vi "sync_issues.vi"(10 "CLZ Issues":string[][](array[string]), 11 "CV Issues":string[][](array[string])) -> (3 "Array":T1[](array[typedef]))   [LabVIEW 2024, in "CLZ_to_ComicVine.lvlib"]
uses:
  CLZ_to_ComicVine.lvlib
  typedefs/issue_match--cluster.ctl
  typedefs/clz_matching_issue--cluster.ctl
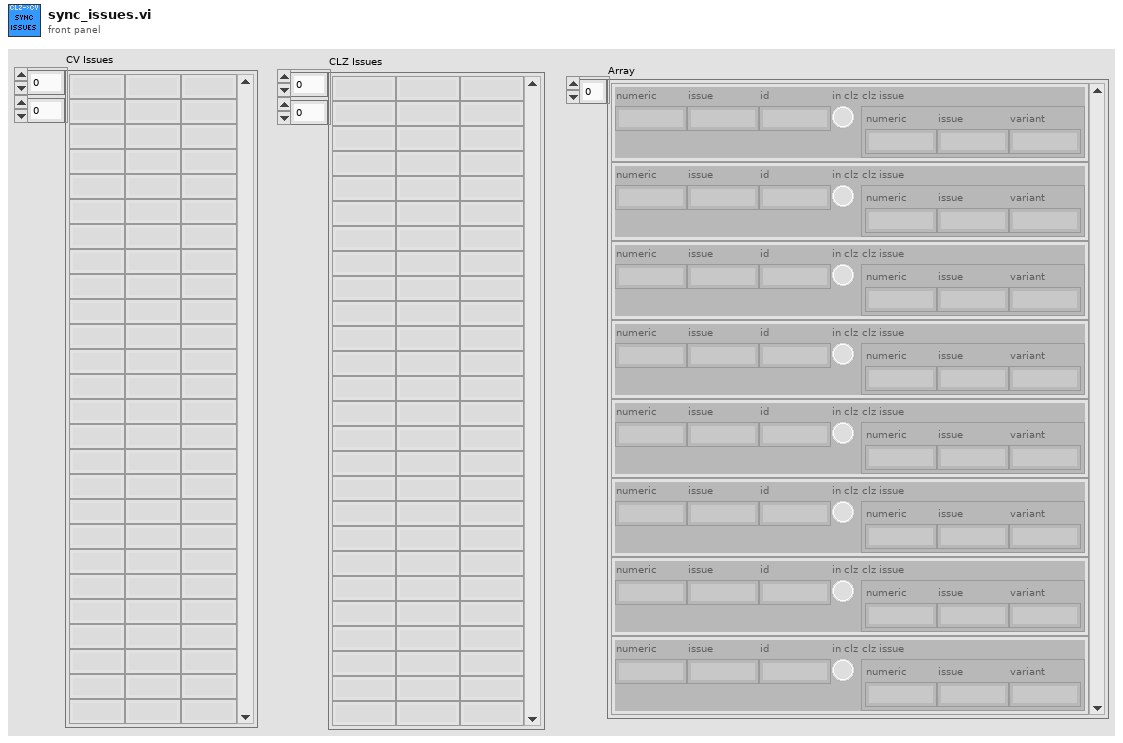
[diagram p1: front panel]
types:
  T1 = typedef "CLZ_to_ComicVine.lvlib/issue_match--cluster.ctl" = cluster{"numeric":string, "issue":string, "id":string, "in clz":bool, "clz issue":T2}
  T2 = typedef "CLZ_to_ComicVine.lvlib/clz_matching_issue--cluster.ctl" = cluster{"numeric":string, "issue":string, "variant":string}
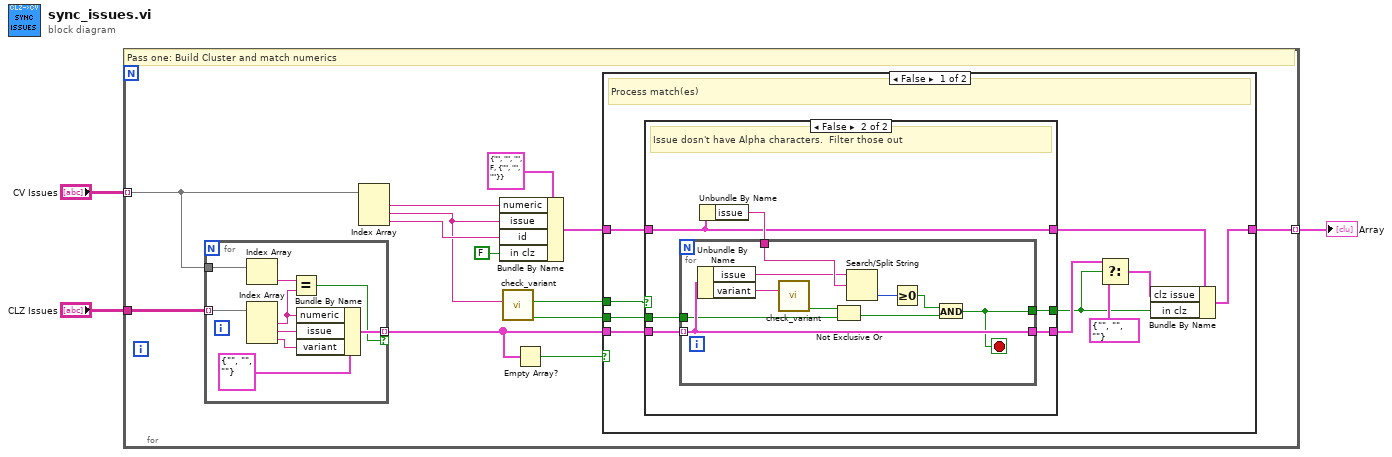
[diagram p0: block diagram]
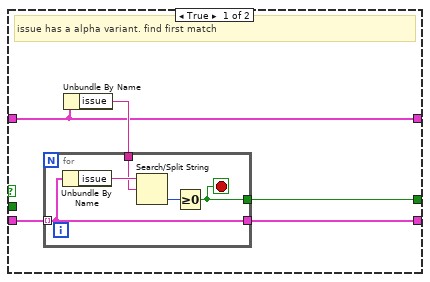
[diagram p2: hidden frame]
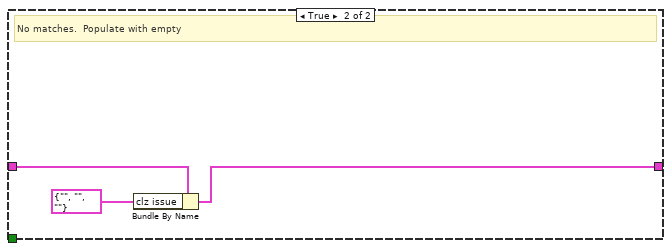
[diagram p3: hidden frame]
diagram:
  n1 = for {
    tunnel: "CV Issues" -> [w14] mode=indexing
    tunnel: "CLZ Issues" -> [w16]
    tunnel: [w5] -> w1 mode=indexing
    # "Pass one: Build Cluster and match numerics"
    n2 = for {
      tunnel: w16 -> [w62] mode=indexing
      tunnel: w14 -> [w64]
      tunnel: [w57] -> w7 mode=indexing if=w56
      n3 = Index Array(array=w64) -> (element=w63:string)  [unwired: 1 in]
      n4 = Index Array(array=w62) -> (element #1=w60:string, element #2=w59:string, element #3=w58:string)  [unwired: 3 in]
      n5 = Equal?(x=w63, y=w60) -> (x = y?=w56:bool)
      n6 = Bundle By Name(cluster=T2 {"numeric"="", "issue"="", "variant"=""} ("clz issue"), "numeric"=w60, "issue"=w59, "variant"=w58) -> (w57:T2)
    }
    n7 = Index Array(array=w14) -> (element #1=w13:string, element #2=w10:string, element #3=w12:string)  [unwired: 3 in]
    n8 = Bundle By Name(cluster=T1 {"numeric"="", "issue"="", "id"="", "in clz"=FALSE, "clz issue"={"numeric"="", "issue"="", "variant"=""}} ("issues"), "numeric"=w13, "issue"=w10, "id"=w12, "in clz"=FALSE) -> (w8:T1)
    n9 = call "check_variant.vi"("String"=w10) -> ("contains decimal"=w4:bool, "contains non-numeric"=w9:bool)  [unwired: 8 in, 1 out]
    n10 = Empty Array?(array=w7) -> (empty?=w6:bool)
    n11 = case shown="False" w6 {
      tunnel: w9 -> [w26 _]
      tunnel: w8 -> [w25 w55]
      tunnel: w7 -> [w24 _]
      tunnel: [w18 w53] -> w5
      tunnel: w4 -> [w17 _]
      frame False {
        # "Process match(es)"
        n12 = case shown="False" w26 {
          tunnel: w24 -> [w31 w42]
          tunnel: w25 -> [w27 w40]
          tunnel: [w27 w40] -> w19
          tunnel: [w28 w39] -> w21
          tunnel: [w29 w38] -> w20
          tunnel: w17 -> [_ w37]
          frame True {
            # "issue has a alpha variant. find first match"
            n13 = Unbundle By Name(w27) -> ("issue"=w30:string)
            n14 = for {
              tunnel: w31 -> [w34] mode=indexing
              tunnel: [w35] -> w29
              tunnel: [w34] -> w28
              tunnel: w30 -> [w32]
              stop <- w35 stop-if-true
              n15 = Unbundle By Name(w34) -> ("issue"=w33:string)
              n16 = Search/Split String(string=w33, search string/char (-)=w32) -> (offset of match=w36:i32)  [unwired: 1 in, 2 out]
              n17 = Greater Or Equal To 0?(x=w36) -> (x >= 0?=w35:bool)
            }
          }
          frame False {
            # "Issue dosn't have Alpha characters.  Filter those out"
            n18 = Unbundle By Name(w40) -> ("issue"=w41:string)
            n19 = for {
              tunnel: w42 -> [w52] mode=indexing
              tunnel: [w43] -> w38
              tunnel: [w52] -> w39
              tunnel: w41 -> [w51]
              tunnel: w37 -> [w46]
              stop <- w43 stop-if-true
              n20 = Unbundle By Name(w52) -> ("issue"=w50:string, "variant"=w48:string)
              n21 = call "check_variant.vi"("String"=w48) -> ("contains decimal"=w47:bool)  [unwired: 8 in, 2 out]
              n22 = Not Exclusive Or(1:w46, 2:w47) -> (0:w44:bool)
              n23 = Search/Split String(string=w50, search string/char (-)=w51) -> (offset of match=w49:i32)  [unwired: 1 in, 2 out]
              n24 = Greater Or Equal To 0?(x=w49) -> (x >= 0?=w45:bool)
              n25 = And(x=w45, y=w44) -> (x .and. y?=w43:bool)
            }
          }
        }
        n26 = Select(t=w21, s=w20, f=T2 {"numeric"="", "issue"="", "variant"=""}) -> (s? t:f=w23:T2)
        n27 = Bundle By Name(cluster=w19, "clz issue"=w23, "in clz"=w20) -> (w18:T1)
      }
      frame True {
        # "No matches.  Populate with empty"
        n28 = Bundle By Name(cluster=w55, "clz issue"=T2 {"numeric"="", "issue"="", "variant"=""}) -> (w53:T1)
      }
    }
  }
  "Array" <- w1
